vi "Module.Window Tasks.vi"(7 "Sys":T1, 8 "error in":errorcluster, 11 "Data1":variant) -> (0 "error out":errorcluster)   [LabVIEW 2024, in "EQMF.lvlib" / "Module Utils.lvlib"]
uses:
  Module Utils.lvlib
  Module Sys Info.ctl
  Config/Stored Controls/Class.SaveCtrls.lvclass
  Event Log/Event Notification/Event Notification.lvclass
  Config/App Data/Class.AppData.lvclass
  Subscription/Subscription.lvclass
  Queues/Q.Element.ctl
  Module.SW Version Info.ctl
  Module Config.ctl
  Module.Working Dirs.ctl
  _Private/Module.Window Task Data.ctl
  Queues/Queue Utils.lvlib
panel:
  # "Name, PN, Version, Note"
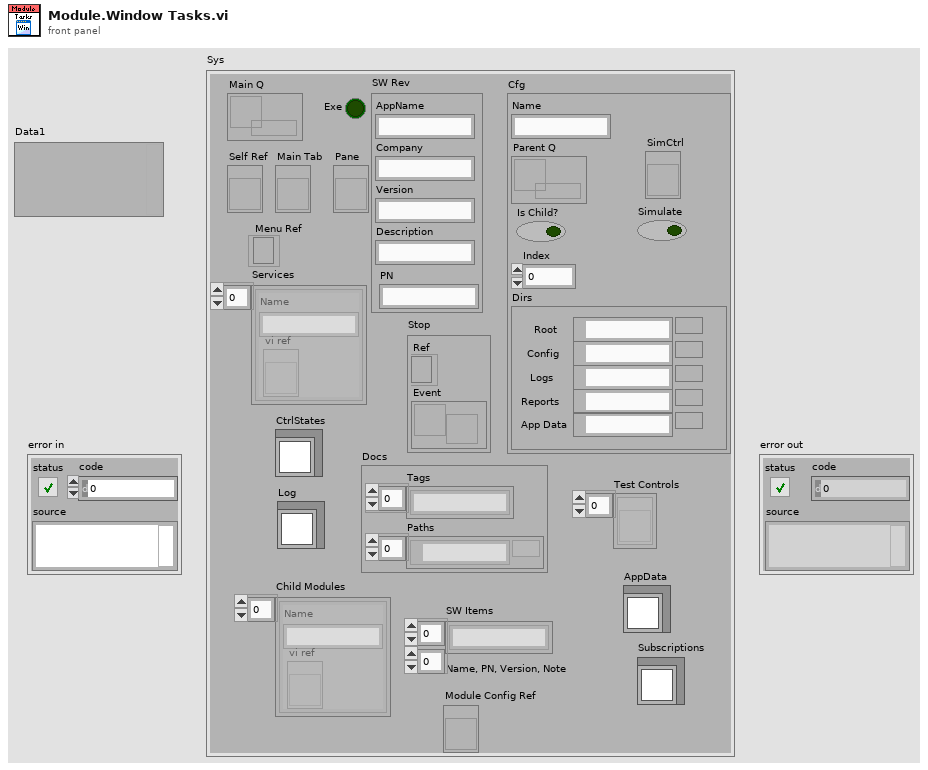
[diagram p1: front panel]
types:
  T1 = typedef "EQMF.lvlib/Module Utils.lvlib/Module Sys Info.ctl" = cluster{"Main Q":refnum<queue>, "Exe":bool, "SW Rev":T2, "Self Ref":refnum<vi>, "Main Tab":refnum<vi>, "Pane":refnum<vi>, "Stop":cluster{"Ref":refnum<event-registration>, "Event":refnum<user-event>}, "Cfg":T3, "Services":cluster{"Name":string, "vi ref":refnum<vi>}[], "Menu Ref":refnum<k9>, "CtrlStates":refnum<class "Class.SaveCtrls.lvclass">, "Docs":cluster{"Tags":string[], "Paths":path[]}, "Log":refnum<class "Event Notification.lvclass">, "Test Controls":refnum<vi>[], "Child Modules":cluster{"Name":string, "vi ref":refnum<vi>}[], "SW Items":string[][], "AppData":refnum<class "Class.AppData.lvclass">, "Subscriptions":refnum<class "Subscription.lvclass">, "Module Config Ref":refnum<vi>}
  T2 = typedef "EQMF.lvlib/Module Utils.lvlib/Module.SW Version Info.ctl" = cluster{"AppName":string, "Company":string, "Version":string, "Description":string, "PN":string}
  T3 = typedef "EQMF.lvlib/Module Utils.lvlib/Module Config.ctl" = cluster{"Name":string, "Parent Q":refnum<queue>, "Is Child?":bool, "Index":i32, "Dirs":T4, "Simulate":bool, "SimCtrl":refnum<vi>}
  T4 = typedef "EQMF.lvlib/Module Utils.lvlib/Module.Working Dirs.ctl" = cluster{"Root":path, "Config":path, "Logs":path, "Reports":path, "App Data":path}
  T5 = typedef "EQMF.lvlib/Module Utils.lvlib/Module.Window Task Data.ctl" = cluster{"Cmd":string, "Data":variant}
  T6 = enum32{"Invalid", "Standard", "Closed", "Hidden", "Minimized", "Maximized"}
  T7 = enum16{"Always On", "Always Off", "Off While Running"}
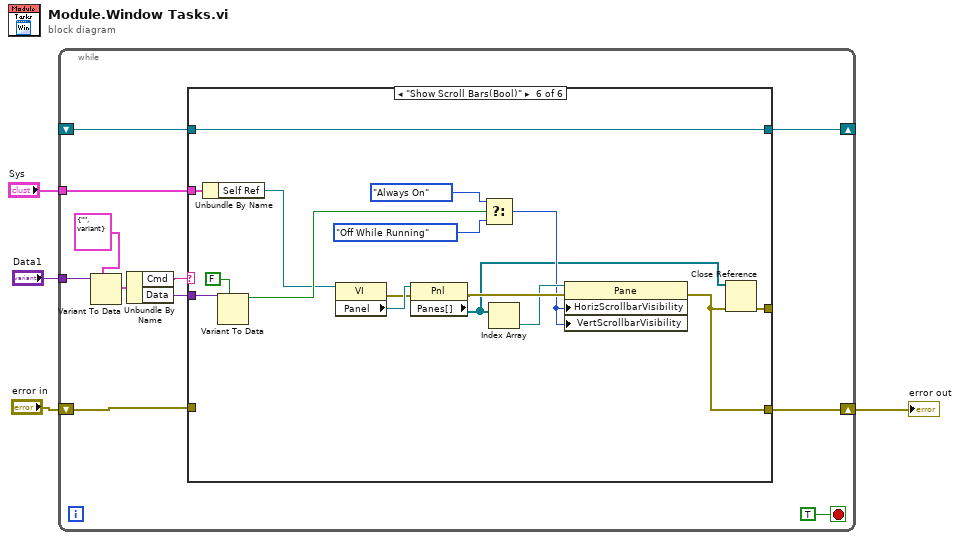
[diagram p0: block diagram]
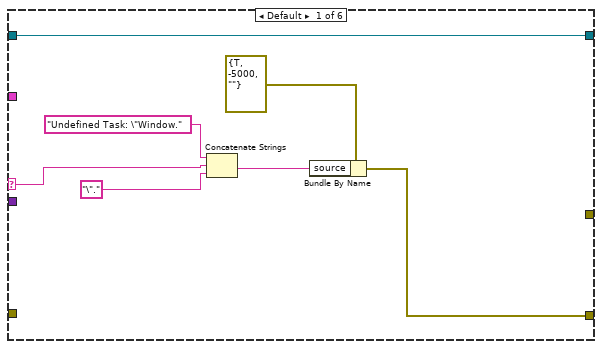
[diagram p2: hidden frame]
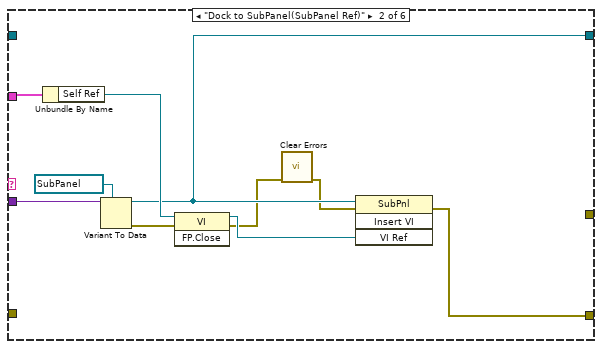
[diagram p3: hidden frame]
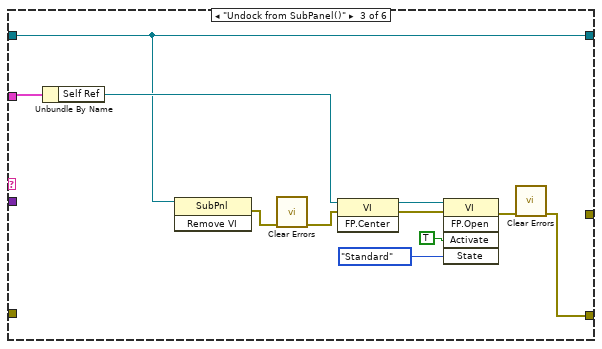
[diagram p4: hidden frame]
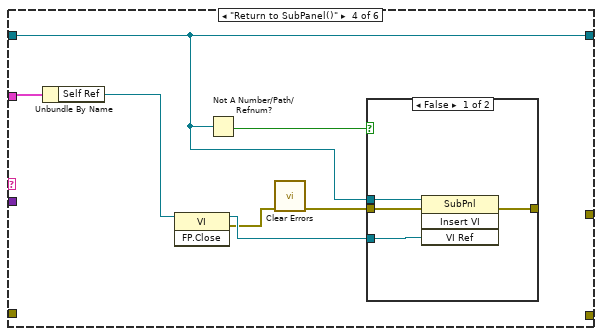
[diagram p5: hidden frame]
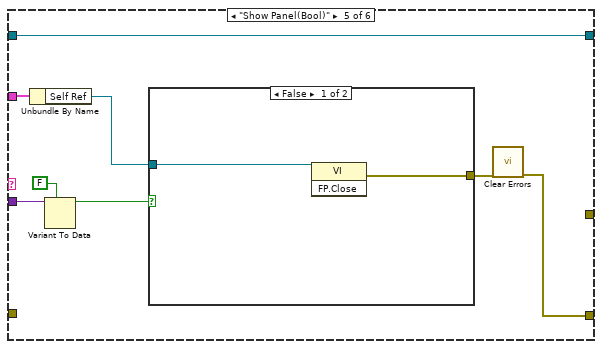
[diagram p7: hidden frame]
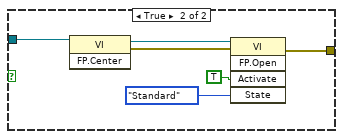
[diagram p8: hidden frame]
diagram:
  n1 = while {
    tunnel: "Sys" -> [w15]
    tunnel: "Data1" -> [w10]
    shift-right: [w13] -> w1
    shift-left: "error in" -> [w14]
    shift-right: [w11] -> _
    shift-left: _ -> [w12]
    stop <- TRUE stop-if-true
    n2 = Variant To Data(type=T5 {"Cmd"="", "Data"=variant}, Variant=w10) -> (data=w8:T5)  [unwired: 1 in, 1 out]
    n3 = Unbundle By Name(w8) -> ("Cmd"=w5:string, "Data"=w7:variant)
    n4 = case shown="\"Show Scroll Bars(Bool)\"" w5 {
      selector: w5 -> [w20 _ _ _ _ _]
      tunnel: w15 -> [_ w32 w43 w50 w61 w75]
      tunnel: w14 -> [_ _ _ _ _ _]
      tunnel: [w18 w26 w33 _ w55 w72] -> w13
      tunnel: w12 -> [w16 _ w35 w45 w62 w86]
      tunnel: [w16 w25 w35 w45 w62 w86] -> w11
      tunnel: w7 -> [_ w29 _ _ w58 w85]
      tunnel: [_ _ _ _ _ w71] -> _
      frame Default {
        n5 = Concatenate Strings("Undefined Task: \"Window.", w20, "\".") -> (w17:string)
        n6 = Bundle By Name(cluster=errorcluster {"status"=TRUE, "code"=-5000, "source"=""} ("error constant"), "source"=w17) -> (w18:errorcluster)
      }
      frame "Dock to SubPanel(SubPanel Ref)" {
        n7 = Unbundle By Name(w32) -> ("Self Ref"=w30:refnum<vi>)
        n8 = Variant To Data(type=refnum<vi> refnum ("reference"), Variant=w29) -> (data=w25:refnum<vi>, error out=w28:errorcluster)  [unwired: 1 in]
        n9 = invoke class="VI" method="FP.Close"(reference=w30, error in=w28) -> (reference out=w27:refnum<vi>, error out=w24:errorcluster)  [unwired: 1 in, 1 out]
        n10 = call <vilib>:"Clear Errors.vi"("error in (no error)"=w24) -> ("error out"=w23:errorcluster)  [unwired: 5 in, 1 out]
        n11 = invoke on="Invoke Node" class="SubPnl" method="Insert VI"(reference=w25, error in=w23, "VI Ref"=w27) -> (error out=w26:errorcluster)  [unwired: 1 in, 3 out]
      }
      frame "Undock from SubPanel()" {
        n12 = Unbundle By Name(w43) -> ("Self Ref"=w37:refnum<vi>)
        n13 = invoke on="Invoke Node" class="SubPnl" method="Remove VI"(reference=w35) -> (error out=w42:errorcluster)  [unwired: 2 in, 2 out]
        n14 = call <vilib>:"Clear Errors.vi"("error in (no error)"=w42) -> ("error out"=w36:errorcluster)  [unwired: 5 in, 1 out]
        n15 = invoke class="VI" method="FP.Center"(reference=w37, error in=w36) -> (reference out=w40:refnum<vi>, error out=w41:errorcluster)  [unwired: 1 in, 1 out]
        n16 = invoke class="VI" method="FP.Open"(reference=w40, error in=w41, "Activate"=TRUE ("Activate?"), "State"=T6."Standard") -> (error out=w34:errorcluster)  [unwired: 1 in, 4 out]
        n17 = call <vilib>:"Clear Errors.vi"("error in (no error)"=w34) -> ("error out"=w33:errorcluster)  [unwired: 5 in, 1 out]
      }
      frame "Return to SubPanel()" {
        n18 = Unbundle By Name(w50) -> ("Self Ref"=w49:refnum<vi>)
        n19 = invoke class="VI" method="FP.Close"(reference=w49) -> (reference out=w48:refnum<vi>, error out=w46:errorcluster)  [unwired: 2 in, 1 out]
        n20 = Not A Number/Path/Refnum?(number/path/refnum=w45) -> (NaN/Path/Refnum?=w44:bool)
        n21 = call <vilib>:"Clear Errors.vi"("error in (no error)"=w46) -> ("error out"=w47:errorcluster)  [unwired: 5 in, 1 out]
        n22 = case shown="False" w44 {
          tunnel: w48 -> [w54 _]
          tunnel: w47 -> [w53 _]
          tunnel: w45 -> [w52 _]
          tunnel: [w51 _] -> _
          frame False {
            n23 = invoke on="Invoke Node" class="SubPnl" method="Insert VI"(reference=w52, error in=w53, "VI Ref"=w54) -> (error out=w51:errorcluster)  [unwired: 1 in, 3 out]
          }
          frame True {
          }
        }
      }
      frame "Show Panel(Bool)" {
        n24 = Unbundle By Name(w61) -> ("Self Ref"=w60:refnum<vi>)
        n25 = Variant To Data(type=FALSE, Variant=w58) -> (data=w57:bool)  [unwired: 1 in, 1 out]
        n26 = case shown="False" w57 {
          tunnel: w60 -> [w64 w66]
          tunnel: [w63 w65] -> w56
          frame False {
            n27 = invoke class="VI" method="FP.Close"(reference=w64) -> (error out=w63:errorcluster)  [unwired: 2 in, 2 out]
          }
          frame True {
            n28 = invoke class="VI" method="FP.Center"(reference=w66) -> (reference out=w69:refnum<vi>, error out=w70:errorcluster)  [unwired: 2 in, 1 out]
            n29 = invoke class="VI" method="FP.Open"(reference=w69, error in=w70, "Activate"=TRUE ("Activate?"), "State"=T6."Standard") -> (error out=w65:errorcluster)  [unwired: 1 in, 4 out]
          }
        }
        n30 = call <vilib>:"Clear Errors.vi"("error in (no error)"=w56) -> ("error out"=w55:errorcluster)  [unwired: 5 in, 1 out]
      }
      frame "Show Scroll Bars(Bool)" {
        n31 = Unbundle By Name(w75) -> ("Self Ref"=w74:refnum<vi>)
        n32 = Variant To Data(type=FALSE, Variant=w85) -> (data=w83:bool)  [unwired: 1 in, 1 out]
        n33 = property class="VI"(reference=w74) -> (error out=w80:errorcluster, "Panel"=w82:refnum<vi>)  [unwired: 1 in, 1 out]
        n34 = property class="Pnl"(reference=w82, error in=w80) -> (error out=w81:errorcluster, "Panes[]"=w73:refnum<vi>[])  [unwired: 1 out]
        n35 = Select(t=T7."Always On" ("Horizontal Scrollbar Visibility"), s=w83, f=T7."Off While Running" ("Horizontal Scrollbar Visibility")) -> (s? t:f=w78:T7)
        n36 = Index Array(array=w73) -> (element=w79:refnum<vi>)  [unwired: 1 in]
        n37 = property class="Pane"(reference=w79, error in=w81, "HorizScrollbarVisibility"=w78, "VertScrollbarVisibility"=w78) -> (error out=w72:errorcluster)  [unwired: 1 out]
        n38 = Close Reference(reference=w73, error in (no error)=w72) -> (error out=w71:errorcluster)
      }
    }
  }
  "error out" <- w1
